vi "uA__daq_Set_diana_uA_Vbat_for_reading.vi"(8 "error in (no error)":errorcluster, 11 "USB DAQ in":tag) -> (0 "error out":errorcluster, 3 "Refnum out":refnum<k21>)   [LabVIEW 2015]
uses:
  <vilib>/DAQmx/create/channels.llb/DAQmx Create Channel (AI-Voltage-Basic).vi
  <vilib>/DAQmx/configure/timing.llb/DAQmx Timing (Sample Clock).vi
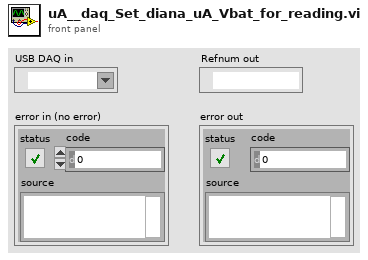
[diagram p1: front panel]
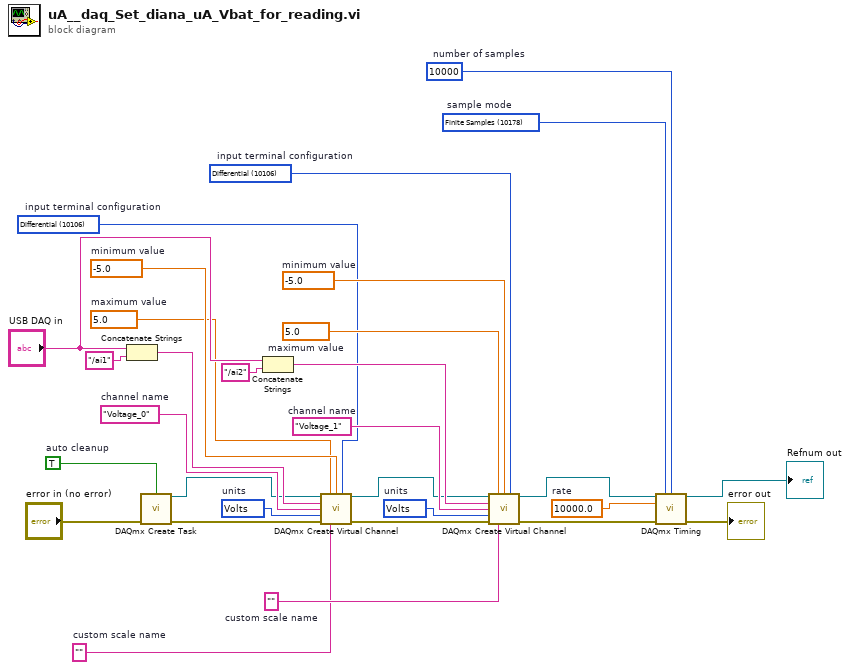
[diagram p0: block diagram]
diagram:
  w22 = 10178 items=["Finite Samples"=10178, "Continuous Samples"=10123, "Hardware Timed Single Point"=12522]  # sample mode
  w21 = 10000  # number of samples
  w20 = 10000.0  # rate
  w18 = 10106 items=["default"=-1, "RSE"=10083, "NRSE"=10078, "Differential"=10106, "Pseudodifferential"=12529]  # input terminal configuration
  w17 = 10348 items=["Volts"=10348, "From Custom Scale"=10065]  # units
  w16 = "Voltage_1"  # channel name
  w14 = ""  # custom scale name
  w13 = -5.0  # minimum value
  w12 = 5.0  # maximum value
  w10 = 10106 items=["default"=-1, "RSE"=10083, "NRSE"=10078, "Differential"=10106, "Pseudodifferential"=12529]  # input terminal configuration
  w9 = 10348 items=["Volts"=10348, "From Custom Scale"=10065]  # units
  w8 = "Voltage_0"  # channel name
  w6 = ""  # custom scale name
  w5 = -5.0  # minimum value
  w4 = 5.0  # maximum value
  w2 = TRUE  # auto cleanup
  n1 = Concatenate Strings("USB DAQ in", "/ai1") -> (w29:string)
  n2 = call <vilib>:"DAQmx Create Task.vi"("auto cleanup"=w2, "error in"="error in (no error)") -> ("task out"=w3:refnum<k21>, "error out"=w1:errorcluster)  [unwired: 12 in]
  n3 = Concatenate Strings("USB DAQ in", "/ai2") -> (w30:string)
  n4 = call-poly <vilib>:"DAQmx Create Virtual Channel.vi"("task in"=w3, "maximum value"=w4, "minimum value"=w5, "input terminal configuration"=w10, "physical channels"=w29, "name to assign"=w8, "units"=w9, "error in"=w1, "custom scale name"=w6) -> ("task out"=w11:refnum<k21>, "error out"=w7:errorcluster)  [unwired: 5 in]
  n5 = call-poly <vilib>:"DAQmx Create Virtual Channel.vi"("task in"=w11, "maximum value"=w12, "minimum value"=w13, "input terminal configuration"=w18, "physical channels"=w30, "name to assign"=w16, "units"=w17, "error in"=w7, "custom scale name"=w14) -> ("task out"=w19:refnum<k21>, "error out"=w15:errorcluster)  [unwired: 5 in]
  n6 = call-poly <vilib>:"DAQmx Timing.vi"("task/channels in"=w19, "sample mode"=w22, "samples per channel"=w21, "rate"=w20, "error in"=w15) -> ("task out"=→"Refnum out":refnum<k21>, "error out"=→"error out":errorcluster)  [unwired: 9 in]
